vi "Write Counter Mode.vi"(8 "error in":errorcluster, 10 "Counter Mode":T1, 11 "MB_TCP session in":refnum<class "MB_Master_TCP.lvclass">) -> (0 "error out":errorcluster, 3 "MB session out":refnum<class "MB_Master_TCP.lvclass">)   [LabVIEW 2024, in "Bronkhorst Flexi-Flow ModbusTCP API.lvlib"]
uses:
  Bronkhorst Flexi-Flow ModbusTCP API.lvlib
  <vilib>/Plasmionique/MB Master/MB_Master_TCP/MB_Master_TCP.lvclass
  Counter Modes--enum.ctl
  PDU Address Char 8-bit Params--ring.ctl
  Write Char Register.vi
  Read Char Register.vi
panel:
  out "Unsigned Char":string
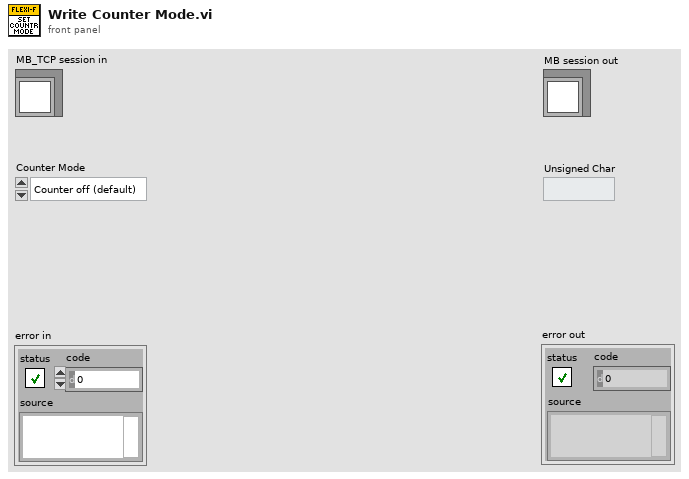
[diagram p1: front panel]
types:
  T1 = typedef "Bronkhorst Flexi-Flow ModbusTCP API.lvlib/Counter Modes--enum.ctl" = enum16{"Counter off (default)", "Counting up continuously", "Counting up until limit reached"}
  T2 = typedef "Bronkhorst Flexi-Flow ModbusTCP API.lvlib/PDU Address Char 8-bit Params--ring.ctl" = u16
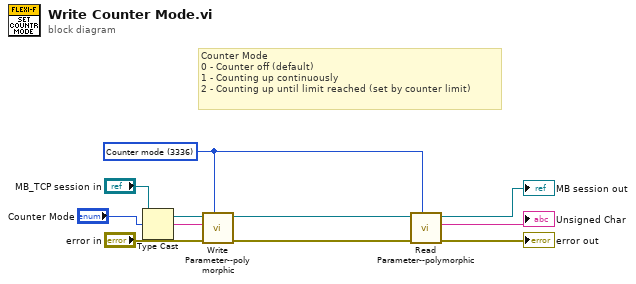
[diagram p0: block diagram]
diagram:
  w1 = T2 3336 items=["Wink"=0, "Control mode"=36, "Alarm mode"=3107, "Alarm setpoint"=3109, "Reset alarm enable"=3113, "Counter unit index"=3330, "Counter setpoint mode"=3333, "Counter mode"=3336, "Reset counter enable"=3337, "Modbus slave address"=4010] ("PDU Address Char 8-bit")
  # "Counter Mode\n0 - Counter off (default)\n1 - Counting up continuously\n2 - Counting up until limit reached (set by counter limit)"
  n1 = Type Cast(x="Counter Mode") -> (*(type *) &x=w2:string)  [unwired: 1 in]
  n2 = call-poly "Write Parameter--polymorphic.vi"("PDU Address Char 8-bit"=w1, "error in"="error in", "Unsigned Char"=w2, "MB_TCP session in"="MB_TCP session in") -> ("error out"=w6:errorcluster, "MB session out"=w8:refnum<class "MB_Master_TCP.lvclass">)  [unwired: 6 in]
  n3 = call-poly "Read Parameter--polymorphic.vi"("PDU Address Char 8-bit"=w1, "error in"=w6, "MB_TCP session in"=w8) -> ("error out"=→"error out":errorcluster, "Unsigned Char"=→"Unsigned Char":string, "MB session out"=→"MB session out":refnum<class "MB_Master_TCP.lvclass">)  [unwired: 6 in]
